vi "MakeDoor.vi"(8 "error in (no error)":errorcluster, 9 "Room 2":refnum<class "Room.lvclass">, 10 "Room 1":refnum<class "Room.lvclass">, 11 "MazeGame in":refnum<class "EnchantedMazeGame.lvclass">) -> (0 "error out":errorcluster, 2 "Door":refnum<class "Door.lvclass">, 3 "MazeGame out":refnum<class "EnchantedMazeGame.lvclass">)   [LabVIEW 2020, in "FactoryMethod.lvlib" / "NoParametrizedFactoryMethod.lvlib" / "EnchantedMazeGame.lvclass"]
uses:
  EnchantedMazeGame.lvclass
  GoFcommonClasses/ConcreteMazeSite/Room/Room.lvclass
  GoFcommonClasses/ConcreteMazeSite/Door/Door.lvclass
  GoFcommonClasses/ConcreteMazeSite/DoorNeedingSpell/DoorNeedingSpell.lvclass
  E:/GitHub/Design-Patterns-GoF_-_NI-LV/Creational/GoFcommonClasses/ConcreteMazeSite/Door/Door.lvclass
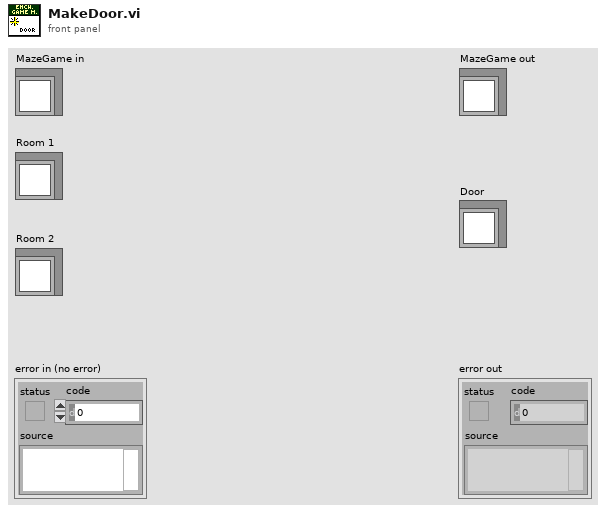
[diagram p1: front panel]
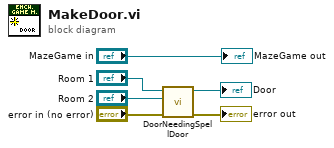
[diagram p0: block diagram]
diagram:
  n1 = call "DoorNeedingSpellDoor.vi"("error in (no error)"="error in (no error)", "Room 2"="Room 2", "Room 1"="Room 1") -> ("error out"=→"error out":errorcluster, "DoorNeedingSpell"=→"Door":refnum<class "DoorNeedingSpell.lvclass">)  [unwired: 7 in]
  "MazeGame out" <- "MazeGame in"
